vi "CSM - Switch Language Tool.vi"() -> ()   [LabVIEW 2017]
doc: "Switch the language of CSM development tools, currently supports Chinese and English."
uses:
  _ui/csm-ui-support.lvlib
  _Shared/CSM Shared.lvlib
panel:
  in  "API Dir":path[](array[path])
  in  "doc dir":path[](array[path])
  in  "options":cluster{"Force?(F)":bool, "Show FP":bool}
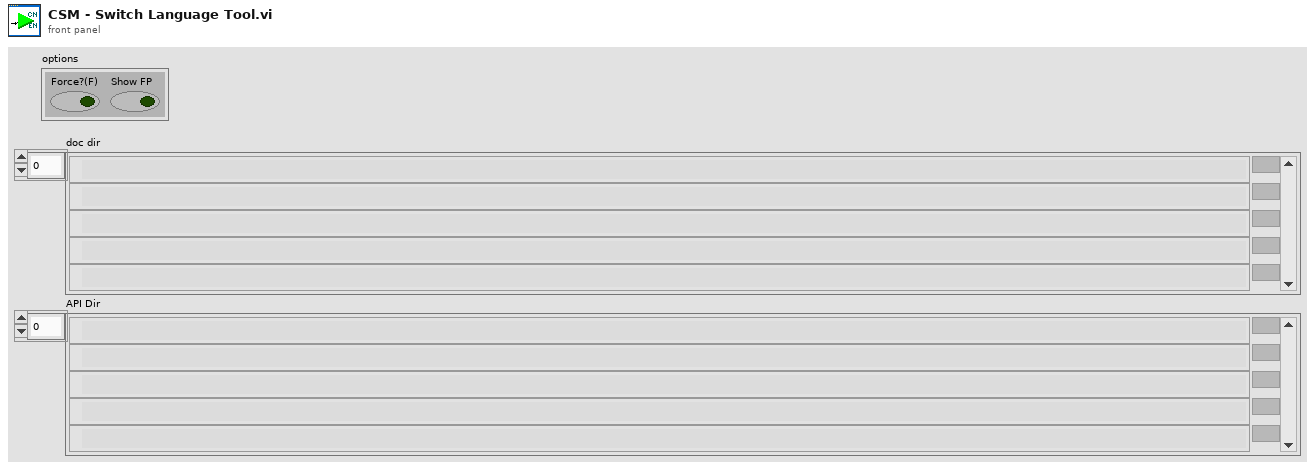
[diagram p1: front panel]
types:
  T1 = enum32{"Invalid", "Standard", "Closed", "Hidden", "Minimized", "Maximized"}
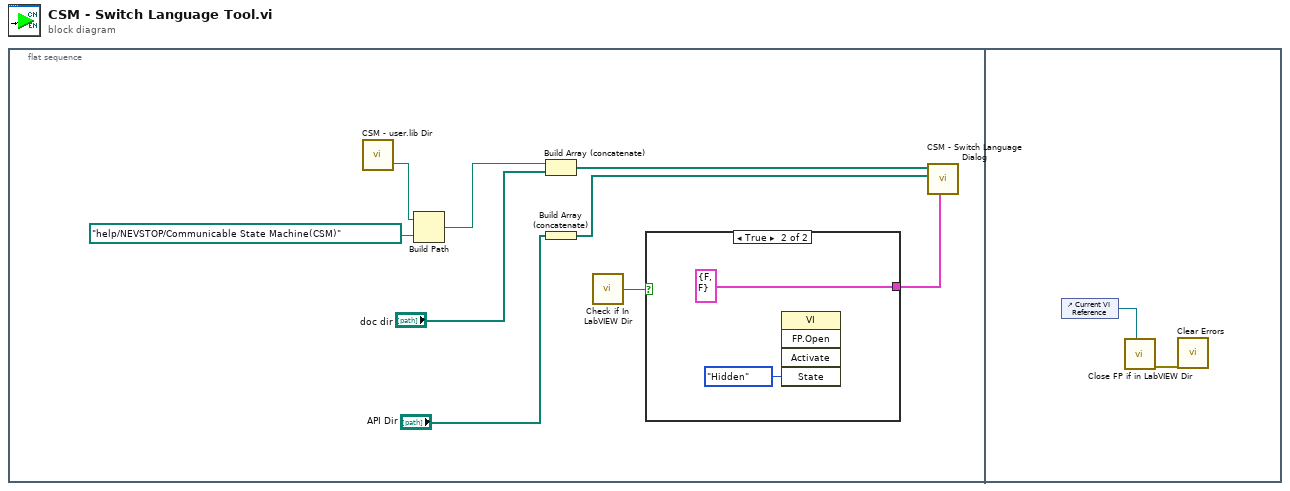
[diagram p0: block diagram]
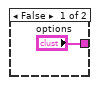
[diagram p2: hidden frame]
diagram:
  n1 = flat-sequence {
    frame #0 {
      n2 = call "CSM - user.lib Dir.vi"() -> ("<LabVIEW>"=w6:path)  [unwired: 2 in, 1 out]
      n3 = Build Path(base path=w6, name or relative path=path "help/NEVSTOP/Communicable State Machine(CSM)") -> (appended path=w3:path)
      n4 = Build Array (concatenate)(w3, "doc dir") -> (w1:path[])
      n5 = Build Array (concatenate)("API Dir") -> (w2:path[])
      n6 = call "Check if In LabVIEW Dir.vi"() -> ("Boolean"=w8:bool)  [unwired: 2 in]
      n7 = case shown="True" w8 {
        tunnel: ["options" cluster{"Force?(F)":bool, "Show FP":bool} {"Force?(F)"=FALSE, "Show FP"=FALSE} ("options")] -> w9
        frame False {
        }
        frame True {
          n8 = invoke class="VI" method="FP.Open"("State"=T1."Hidden") -> ()  [unwired: 4 in, 5 out]
        }
      }
      n9 = call "CSM - Switch Language Dialog.vi"("options"=w9, "API Dir"=w2, "doc dir"=w1) -> ()  [unwired: 9 in]
    }
    frame #1 {
      n10 = control-ref of="Current VI Reference"() -> (w13:refnum<vi>)
      n11 = call "Close FP if in LabVIEW Dir.vi"("VI Refnum"=w13) -> ("Error out"=w14:errorcluster)  [unwired: 10 in]
      n12 = call <vilib>:"Clear Errors.vi"("error in (no error)"=w14) -> ()  [unwired: 5 in, 2 out]
    }
  }
